vi "EMV Basic Cold Water Check.vi"(6 "Cold Water Supply Temperature in":dbl, 8 "error in (no error)":errorcluster, 9 "T7_DELTA_INDICATING_FLOW":dbl, 11 "Current T7 Temperatures in":dbl[](array[numeric])) -> (0 "error out":errorcluster, 3 "Current T7 Temperatures out":dbl[](array[numeric]), 5 "Basic Cold Water Check":bool)   [LabVIEW 2020]
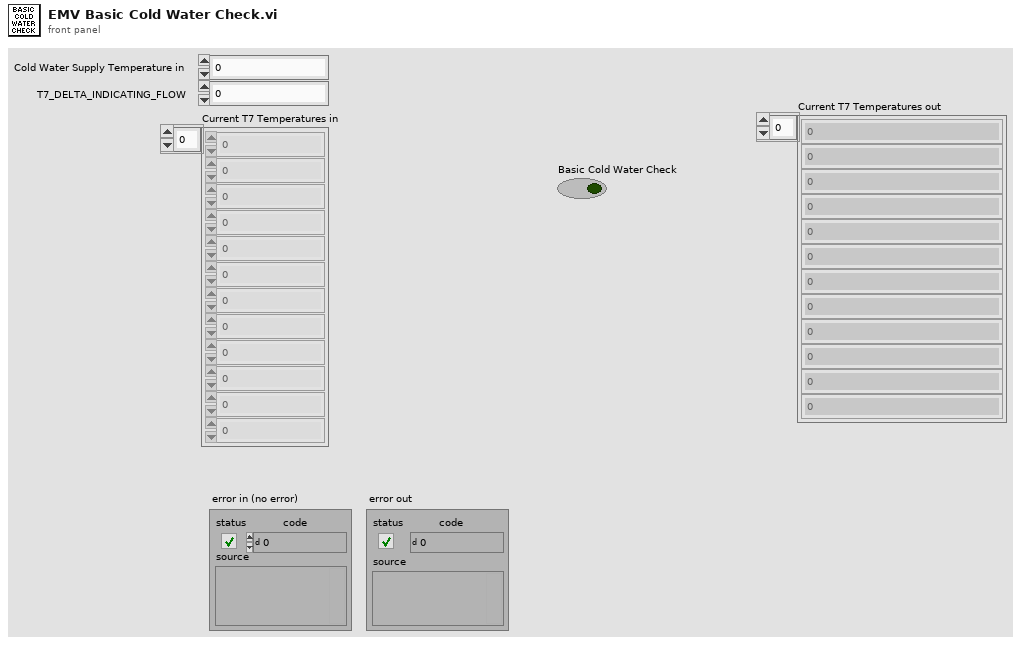
[diagram p1: front panel]
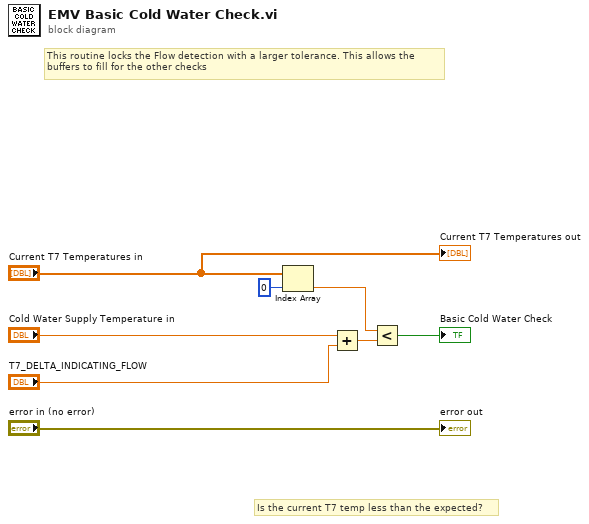
[diagram p0: block diagram]
diagram:
  # "This routine locks the Flow detection with a larger tolerance. This allows the\nbuffers to fill for the other checks"
  # "Is the current T7 temp less than the expected?"
  n1 = Index Array(array="Current T7 Temperatures in", index=0) -> (element=w5:dbl)
  n2 = Add(x="Cold Water Supply Temperature in", y="T7_DELTA_INDICATING_FLOW") -> (x+y=w2:dbl)
  n3 = Less?(x=w5, y=w2) -> (x < y?=→"Basic Cold Water Check":bool)
  "Current T7 Temperatures out" <- "Current T7 Temperatures in"
  "error out" <- "error in (no error)"
